vi "home.vi"   [LabVIEW 2018]
uses:
  <vilib>/MediaMongrels Ltd/WebSockets/WebSockets/WebSocket Client/WebSocket Client.lvclass
  D:/software_setup/National Instruments/LabVIEW 2018/vi.lib/MediaMongrels Ltd/WebSockets/WebSockets/WebSocket/WebSocket.lvclass
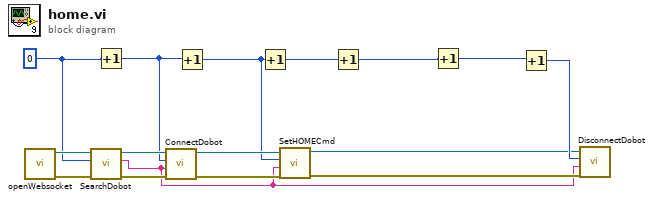
[diagram p0: block diagram]
diagram:
  w12 = 0 ("id")
  n1 = call <vilib>:"openWebsocket.vi"() -> ("error out"=w14:errorcluster, "WebSocket Client out"=w16:refnum<class "WebSocket Client.lvclass">)  [unwired: 10 in]
  n2 = call <vilib>:"SearchDobot.vi"("error in (no error)"=w14, "id"=w12, "WebSocket in"=w16) -> ("error out"=w13:errorcluster, "portName"=w1:string, "WebSocket out"=w15:refnum<class "WebSocket Client.lvclass">)  [unwired: 6 in]
  n3 = Increment(x=w12) -> (x+1=w11:i32)
  n4 = call <vilib>:"ConnectDobot.vi"("error in (no error)"=w13, "portName"=w1, "id"=w11, "WebSocket in"=w15) -> ("error out"=w5:errorcluster, "WebSocket out"=w6:refnum<class "WebSocket Client.lvclass">)  [unwired: 5 in, 1 out]
  n5 = Increment(x=w11) -> (x+1=w2:i32)
  n6 = Increment(x=w2) -> (x+1=w9:i32)
  n7 = call <vilib>:"SetHOMECmd.vi"("error in (no error)"=w5, "portName"=w1, "id"=w2, "WebSocket in"=w6) -> ("error out"=w3:errorcluster, "WebSocket out"=w4:refnum<class "WebSocket Client.lvclass">)  [unwired: 5 in, 1 out]
  n8 = Increment(x=w9) -> (x+1=w8:i32)
  n9 = Increment(x=w8) -> (x+1=w7:i32)
  n10 = Increment(x=w7) -> (x+1=w10:i32)
  n11 = call <vilib>:"DisconnectDobot.vi"("error in (no error)"=w3, "portName"=w1, "id"=w10, "WebSocket in"=w4) -> ()  [unwired: 5 in, 3 out]
